vi "LoadControlPanel.vi"(8 "error in (no error)":errorcluster, 10 "Actor In":refnum<class "Actor.lvclass">, 11 "DemoStage in":refnum<class "DemoStage.lvclass">) -> (0 "error out":errorcluster, 3 "DemoStage out":refnum<class "DemoStage.lvclass">)   [LabVIEW 2020, in "DemoStage.lvlib" / "DemoStage.lvclass"]
uses:
  DemoStage.lvclass
  <vilib>/ActorFramework/Actor/Actor.lvclass
  ViewController/TripleAxisStageController/TriaxesStageController.lvclass
  C:/Program Files/National Instruments/LabVIEW 2020/vi.lib/ActorFramework/Actor/Actor.lvclass
  Hardware Abstraction Layer/Component/Stage/Stage/Stage.lvclass
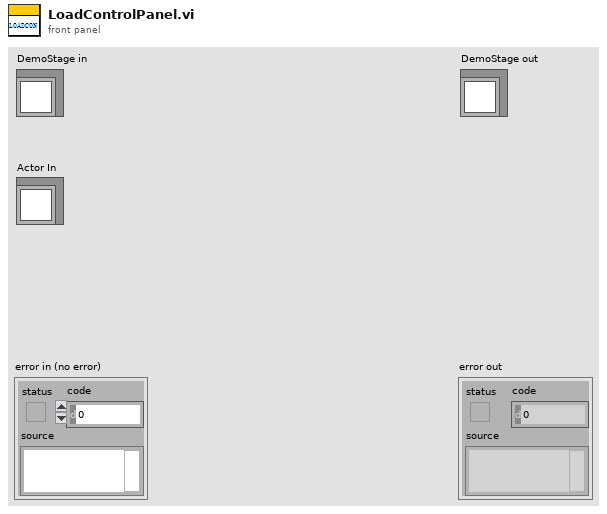
[diagram p1: front panel]
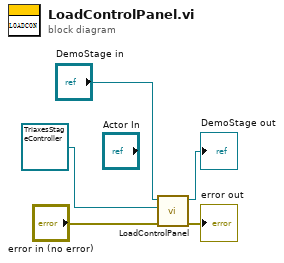
[diagram p0: block diagram]
diagram:
  n1 = call-parent "LoadControlPanel.vi"("error in (no error)"="error in (no error)", "Actor In"=refnum<class "TriaxesStageController.lvclass"> refnum ("TripleAxisStageController.lvlib:TripleAxisStageController.lvclass"), "GRMActor in"="DemoStage in") -> ("error out"=→"error out":errorcluster, "GRMActor out"=→"DemoStage out":refnum<class "DemoStage.lvclass">)  [unwired: 7 in]
